vi "[SubVI]Encoder_Position.vi"(5 "SPI Reference In in":T1 {"SPI Configuration"."Frame Length" min=1 max=16}) -> (0 "Left Theta":dbl, 1 "Right Theta":dbl, 2 "SPI Reference In out":T1 {"SPI Configuration"."Frame Length" min=1 max=16}, 3 "Left Raw":u16, 4 "Right Raw":u16)   [LabVIEW 2019]
uses:
  <vilib>/myRIO/Instrument Drivers/Onboard IO/SPI/typedefs/SPI Reference.ctl
  <vilib>/myRIO/Common/Instrument Driver Framework/Utilities/typedefs/myRIO Generic Hardware Reference.ctl
  <vilib>/myRIO/Common/Instrument Driver Framework/Utilities/typedefs/Hardware Version Enum.ctl
  <vilib>/myRIO/Common/Instrument Driver Framework/Utilities/typedefs/myRIO v1.0 Reference.ctl
  <vilib>/myRIO/Common/Instrument Driver Framework/Utilities/typedefs/Generic FPGA Reference.ctl
  <vilib>/myRIO/Common/Instrument Driver Framework/myRIO v1.0/SPI/typedefs/SPI Channels Enum.ctl
  <vilib>/myRIO/Instrument Drivers/Onboard IO/SPI/typedefs/SPI Configuration.ctl
  <vilib>/myRIO/Common/Instrument Driver Framework/myRIO v1.0/SPI/typedefs/SPI Clock Phase.ctl
  <vilib>/myRIO/Common/Instrument Driver Framework/myRIO v1.0/SPI/typedefs/SPI Clock Polarity.ctl
  <vilib>/myRIO/Common/Instrument Driver Framework/myRIO v1.0/SPI/typedefs/SPI Data Direction.ctl
  <vilib>/myRIO/Common/Instrument Driver Framework/myRIO v1.0/SPI/typedefs/SPI Frame Length.ctl
  <vilib>/myRIO/Instrument Drivers/Onboard IO/DIO/typedefs/DIO Reference.ctl
  <vilib>/myRIO/Common/Instrument Driver Framework/myRIO v1.0/DIO/typedefs/DIO Channels List.ctl
  <vilib>/myRIO/Common/Instrument Driver Framework/myRIO v1.0/DIO/typedefs/DIO Channels Enum.ctl
  <vilib>/userdefined/High Color/nirio_resource_hc.ctl
  <vilib>/myRIO/Common/Instrument Driver Framework/Utilities/vis/Is FPGA Ref Available.vi
  <vilib>/myRIO/Common/Instrument Driver Framework/myRIO v1.0/DIO/vis/myRIO v1.1 Open DIO.vi
  <vilib>/myRIO/Instrument Drivers/Onboard IO/DIO/vis/Write.vi
  <vilib>/myRIO/Common/Instrument Driver Framework/Utilities/vis/Validate Channels.vi
  <vilib>/myRIO/Common/Instrument Driver Framework/myRIO v1.0/DIO/vis/myRIO v1.0 Reserve DIO.vi
  <vilib>/myRIO/Instrument Drivers/Onboard IO/SPI/vis/Write Read.vi
  <vilib>/myRIO/Common/Instrument Driver Framework/myRIO v1.0/Resource Manager/vis/myRIO v1.0 Reserve Channel List.vi
  <vilib>/myRIO/Common/Instrument Driver Framework/myRIO v1.0/DIO/vis/myRIO v1.0 Build MUX Configuration DIO.vi
  <vilib>/myRIO/Common/Instrument Driver Framework/myRIO v1.0/Resource Manager/vis/myRIO v1.0 Reserve Channel.vi
  <vilib>/myRIO/Common/Instrument Driver Framework/myRIO v1.0/Resource Manager/vis/myRIO v1.0 Unreserve Channel.vi
  <vilib>/myRIO/Common/Instrument Driver Framework/myRIO v1.0/Resource Manager/vis/myRIO v1.0 Create Configuration List.vi
  <vilib>/myRIO/Common/Instrument Driver Framework/myRIO v1.0/Resource Manager/vis/myRIO v1.0 Build Mutex Name.vi
  <vilib>/Utility/VariantDataType/GetNumericInfo.vi
  <vilib>/Utility/error.llb/Error Cluster From Error Code.vi
  <vilib>/myRIO/Common/Instrument Driver Framework/myRIO v1.0/myRIO v1.1 Open.vi
  <vilib>/myRIO/Common/Instrument Driver Framework/Utilities/vis/IO Manager.vi
  <vilib>/myRIO/Common/Instrument Driver Framework/Utilities/vis/Configuration Manager.vi
  <vilib>/myRIO/Common/Instrument Driver Framework/myRIO v1.0/Resource Manager/vis/myRIO v1.0 Configure IO.vi
  <vilib>/myRIO/Common/Instrument Driver Framework/myRIO v1.0/myRIO v1.0 Close.vi
  <vilib>/myRIO/Common/Instrument Driver Framework/myRIO v1.0/DIO/vis/myRIO v1.0 Write DIO.vi
  <vilib>/myRIO/Common/Instrument Driver Framework/myRIO v1.0/SPI/vis/myRIO v1.0 Write Read SPI.vi
  <vilib>/myRIO/Express VI/Onboard IO/DO/DO Express VI.xnode
  <vilib>/myRIO/Instrument Drivers/Onboard IO/DIO/vis/myRIO DIO Open.xnode
  <vilib>/myRIO/Instrument Drivers/Onboard IO/DIO/DIO.lvlib
  <vilib>/myRIO/Instrument Drivers/Onboard IO/SPI/SPI.lvlib
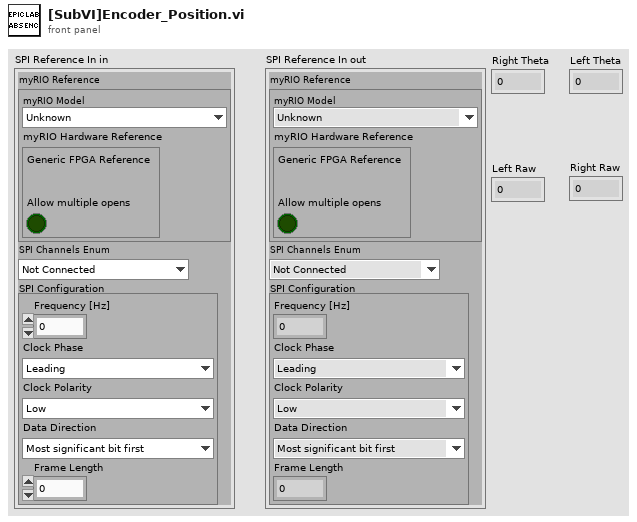
[diagram p1: front panel]
types:
  T1 = typedef "SPI.lvlib/SPI Reference.ctl" = cluster{"myRIO Reference":T2, "SPI Channels Enum":T6, "SPI Configuration":T7}
  T2 = typedef "myRIO Generic Hardware Reference.ctl" = cluster{"myRIO Model":T3, "myRIO Hardware Reference":T4}
  T3 = typedef "Hardware Version Enum.ctl" = enum16{"Unknown", "myRIO-1900", "myRIO-1950", "roboRIO", "NI ELVIS RIO CM", "ELVIS III"}
  T4 = typedef "myRIO v1.0 Reference.ctl" = cluster{"Generic FPGA Reference":T5, "Allow multiple opens":bool}
  T5 = typedef "Generic FPGA Reference.ctl" = refnum<k20>
  T6 = typedef "SPI Channels Enum.ctl" = enum16{"Not Connected", "A/SPI", "B/SPI", "SPI/SPI"}
  T7 = typedef "SPI.lvlib/SPI Configuration.ctl" = cluster{"Frequency [Hz]":dbl, "Clock Phase":T8, "Clock Polarity":T9, "Data Direction":T10, "Frame Length":T11}
  T8 = typedef "SPI Clock Phase.ctl" = enum8{"Leading", "Trailing"}
  T9 = typedef "SPI Clock Polarity.ctl" = enum8{"Low", "High"}
  T10 = typedef "SPI Data Direction.ctl" = enum8{"Most significant bit first", "Least significant bit first"}
  T11 = typedef "SPI Frame Length.ctl" = u8
  T12 = typedef "DIO.lvlib/DIO Reference.ctl" = cluster{"myRIO Reference":T2, "DIO Channels List":T13}
  T13 = typedef "DIO Channels List.ctl" = T14[]
  T14 = typedef "DIO Channels Enum.ctl" = enum16{"Not Connected", "C/DIO0", "C/DIO1", "C/DIO2", "C/DIO3", "C/DIO4", "C/DIO5", "C/DIO6", "C/DIO7", "A/DIO0", "A/DIO1", "A/DIO2", "A/DIO3", "A/DIO4", "A/DIO5", "A/DIO6", "A/DIO7", "A/DIO8", "A/DIO9", "A/DIO10", "A/DIO11", "A/DIO12", "A/DIO13", "A/DIO14", "A/DIO15", "A/DIO16", "A/DIO17", "A/DIO18", "A/DIO19", "B/DIO0", "B/DIO1", "B/DIO2", "B/DIO3", "B/DIO4", "B/DIO5", "B/DIO6", "B/DIO7", "B/DIO8", "B/DIO9", "B/DIO10", "B/DIO11", "B/DIO12", "B/DIO13", "B/DIO14", "B/DIO15", "B/DIO16", "B/DIO17", "B/DIO18", "B/DIO19", "LED0", "LED1", "LED2", "LED3", "Button0", "DIO/DIO0", "DIO/DIO1", "DIO/DIO2", "DIO/DIO3", "DIO/DIO4", "DIO/DIO5", "DIO/DIO6", "DIO/DIO7", "DIO/DIO8", "DIO/DIO9", "SPI/CS0", "SPI/CS1", "SPI/CS2", "SPI/CS3", "LED RADIO (Green)", "LED RADIO (Red)", "LED COMM (Green)", "LED COMM (Red)", "LED MODE (Green)", "LED MODE (Red)"}
  T15 = typedef "nirio_resource_hc.ctl" = tag
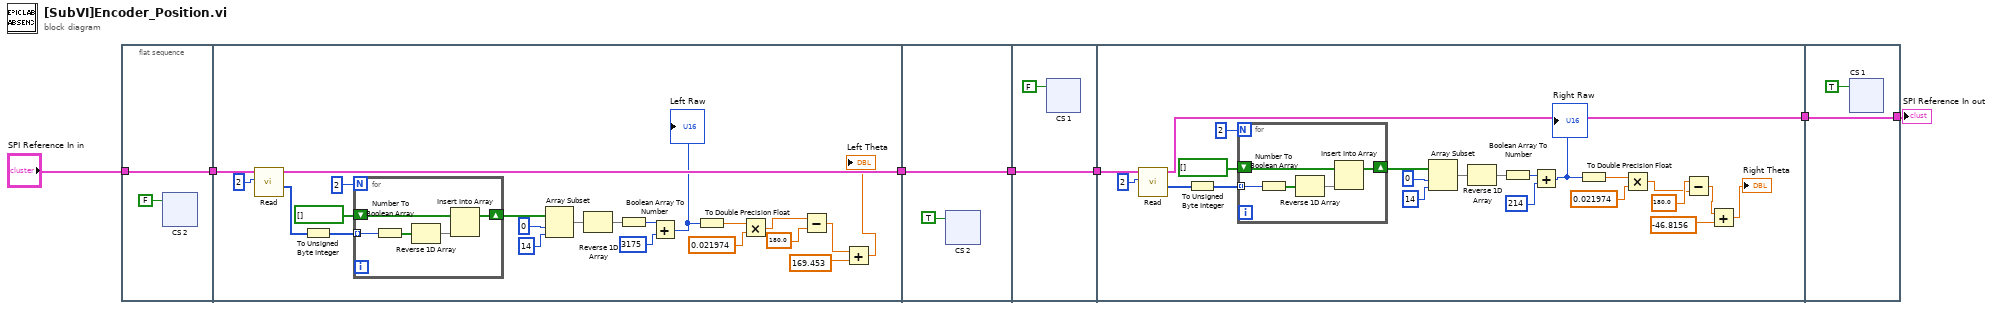
[diagram p0: block diagram]
diagram:
  n1 = flat-sequence {
    tunnel: [w9] -> w6
    tunnel: "SPI Reference In in" -> [w9]
    tunnel: w6 -> [w57]
    tunnel: [w56] -> w2
    tunnel: w2 -> [w73]
    tunnel: [w73] -> w1
    tunnel: w1 -> [w110]
    tunnel: [w110] -> w5
    tunnel: w5 -> [w161]
    tunnel: [w160] -> w4
    tunnel: [w174] -> w3
    tunnel: w4 -> [w174]
    frame #0 {
      n2 = xnode "CS 2"("A/DIO15 (Pin 34)"=FALSE ("A/DIO1 (Pin 13)")) -> ()  [unwired: 1 in, 1 out]
    }
    frame #1 {
      n3 = call <vilib>:"Read.vi"("Frame Count"=u32 2, "SPI Ref In"=w57) -> ("Frames Read"=w58:u16[], "SPI Ref Out"=w56:T1)  [unwired: 6 in, 1 out]
      n4 = To Unsigned Byte Integer(number=w58) -> (unsigned 8bit integer=w66:u8[])
      n5 = for {
        N: 2 -> [_]
        tunnel: w66 -> [w71] mode=indexing
        shift-right: [w69] -> w59
        shift-left: bool[] [] -> [w70]
        n6 = Number To Boolean Array(number=w71) -> (Boolean array=w68:bool[])
        n7 = Reverse 1D Array(array=w68) -> (reversed array=w67:bool[])
        n8 = Insert Into Array(array=w70, new element=w67) -> (w69:bool[])  [unwired: 1 in]
      }
      n9 = Array Subset(array=w59, index=0, length=14) -> (w60:bool[])
      n10 = Reverse 1D Array(array=w60) -> (reversed array=w61:bool[])
      n11 = Boolean Array To Number(Boolean array=w61) -> (number=w50:u16)
      n12 = Add(x=w50, y=u16 3175) -> (x+y=w51:u16)
      "Left Raw" <- w51
      n13 = To Double Precision Float(number=w51) -> (double precision float=w53:dbl)
      n14 = Multiply(x=w53, y=0.021974) -> (x*y=w45:dbl)
      n15 = Subtract(x=w45, y=180.0 ("x")) -> (x-y=w48:dbl)
      n16 = Add(x=w48, y=169.453 ("x")) -> (x+y=→"Left Theta":dbl)
    }
    frame #2 {
      n17 = xnode "CS 2"("A/DIO15 (Pin 34)"=TRUE ("A/DIO1 (Pin 13)")) -> ()  [unwired: 1 in, 1 out]
    }
    frame #3 {
      n18 = xnode "CS 1"("A/DIO14 (Pin 32)"=FALSE ("A/DIO2 (Pin 15)")) -> ()  [unwired: 1 in, 1 out]
    }
    frame #4 {
      n19 = call <vilib>:"Read.vi"("Frame Count"=u32 2, "SPI Ref In"=w161) -> ("Frames Read"=w163:u16[], "SPI Ref Out"=w160:T1)  [unwired: 6 in, 1 out]
      n20 = To Unsigned Byte Integer(number=w163) -> (unsigned 8bit integer=w157:u8[])
      n21 = for {
        N: 2 -> [_]
        shift-right: [w169] -> w158
        shift-left: bool[] [] -> [w170]
        tunnel: w157 -> [w168] mode=indexing
        n22 = Number To Boolean Array(number=w168) -> (Boolean array=w172:bool[])
        n23 = Reverse 1D Array(array=w172) -> (reversed array=w171:bool[])
        n24 = Insert Into Array(array=w170, new element=w171) -> (w169:bool[])  [unwired: 1 in]
      }
      n25 = Array Subset(array=w158, index=0, length=14) -> (w164:bool[])
      n26 = Reverse 1D Array(array=w164) -> (reversed array=w165:bool[])
      n27 = Boolean Array To Number(Boolean array=w165) -> (number=w153:u16)
      n28 = Add(x=w153, y=u16 214) -> (x+y=w152:u16)
      "Right Raw" <- w152
      n29 = To Double Precision Float(number=w152) -> (double precision float=w155:dbl)
      n30 = Multiply(x=w155, y=0.021974) -> (x*y=w146:dbl)
      n31 = Subtract(x=180.0 ("y"), y=w146) -> (x-y=w149:dbl)
      n32 = Add(x=w149, y=-46.8156 ("x")) -> (x+y=→"Right Theta":dbl)
    }
    frame #5 {
      n33 = xnode "CS 1"("A/DIO14 (Pin 32)"=TRUE ("A/DIO2 (Pin 15)")) -> ()  [unwired: 1 in, 1 out]
    }
  }
  "SPI Reference In out" <- w3
